vi "tStat2021_V3-19-04-2021.vi"() -> ()   [LabVIEW 2016]
doc: "This VI was designed to demonstrate typical usage of sub VIs containing the more common 335 functions. The VI Initializes the instrument, allows the user to determine if heater output control parameters and setpoint values are sent, takes a single sensor reading, and then closes the instrument."
uses:
  <instrlib>/Lake Shore 335/Public/Data/Sensor Data (Single Reading).vi
  <instrlib>/Lake Shore 335/Lake Shore 335.lvlib
panel:
  out "Ramping On":bool
  out "Ramping Active":bool
  out "Ramp Rate":dbl format="%.1f"
  out "Setpoint":dbl format="%.4f"
  in  "Ramp Rate (0.0)":dbl format="%.1f"
  in  "OK Button 2":bool
  in  "Mode 2":enum32{"Radio Selection 1", "Radio Selection 2"}(radio)
  in  "ШТОК 2":T1(radio)
  in  "Manual Output (0.00 %) 2":dbl format="%.2f"
  in  "Setpoint (0.0000) 2":dbl format="%.4f"
  out "x .and. y?":bool[](array[boolean])
  in  "Manual Output (0.00 %)":dbl format="%.2f"
  in  "Mode":enum32{"Radio Selection 1", "Radio Selection 2"}(radio)
  out "Температура в криоголовке":cluster{"Y":dbl[], "Y":dbl[]}[](graph)
  out "ТЕМПЕРАТУРА В КРИОГОЛОВКЕ":dbl format="%.4f"
  in  "Graph":bool
  out "Current":cluster{"Y":dbl[], "Y":dbl[]}[](graph)
  out "Temperature":cluster{"Y":dbl[], "Y":dbl[]}[](graph)
  in  "ШТОК":T1(radio)
  in  "Exit":bool
  out "Sensor Data":dbl format="%.4f"
  out "Heater power":dbl(graph)
  out "Temperature":dbl(graph)
  in  "Set":bool
  in  "Setpoint (0.0000)":dbl format="%.4f"
  # "Задать Ramping"
  # "Задавать при режиме Open Loop"
  # "Температуру на кpиоголовке"
  # "K/min"
  # "Температуру на кpиоголовке"
  # "(c) 2021 Vladimir Z Inc.  ALL RIGHTS RESERVED."
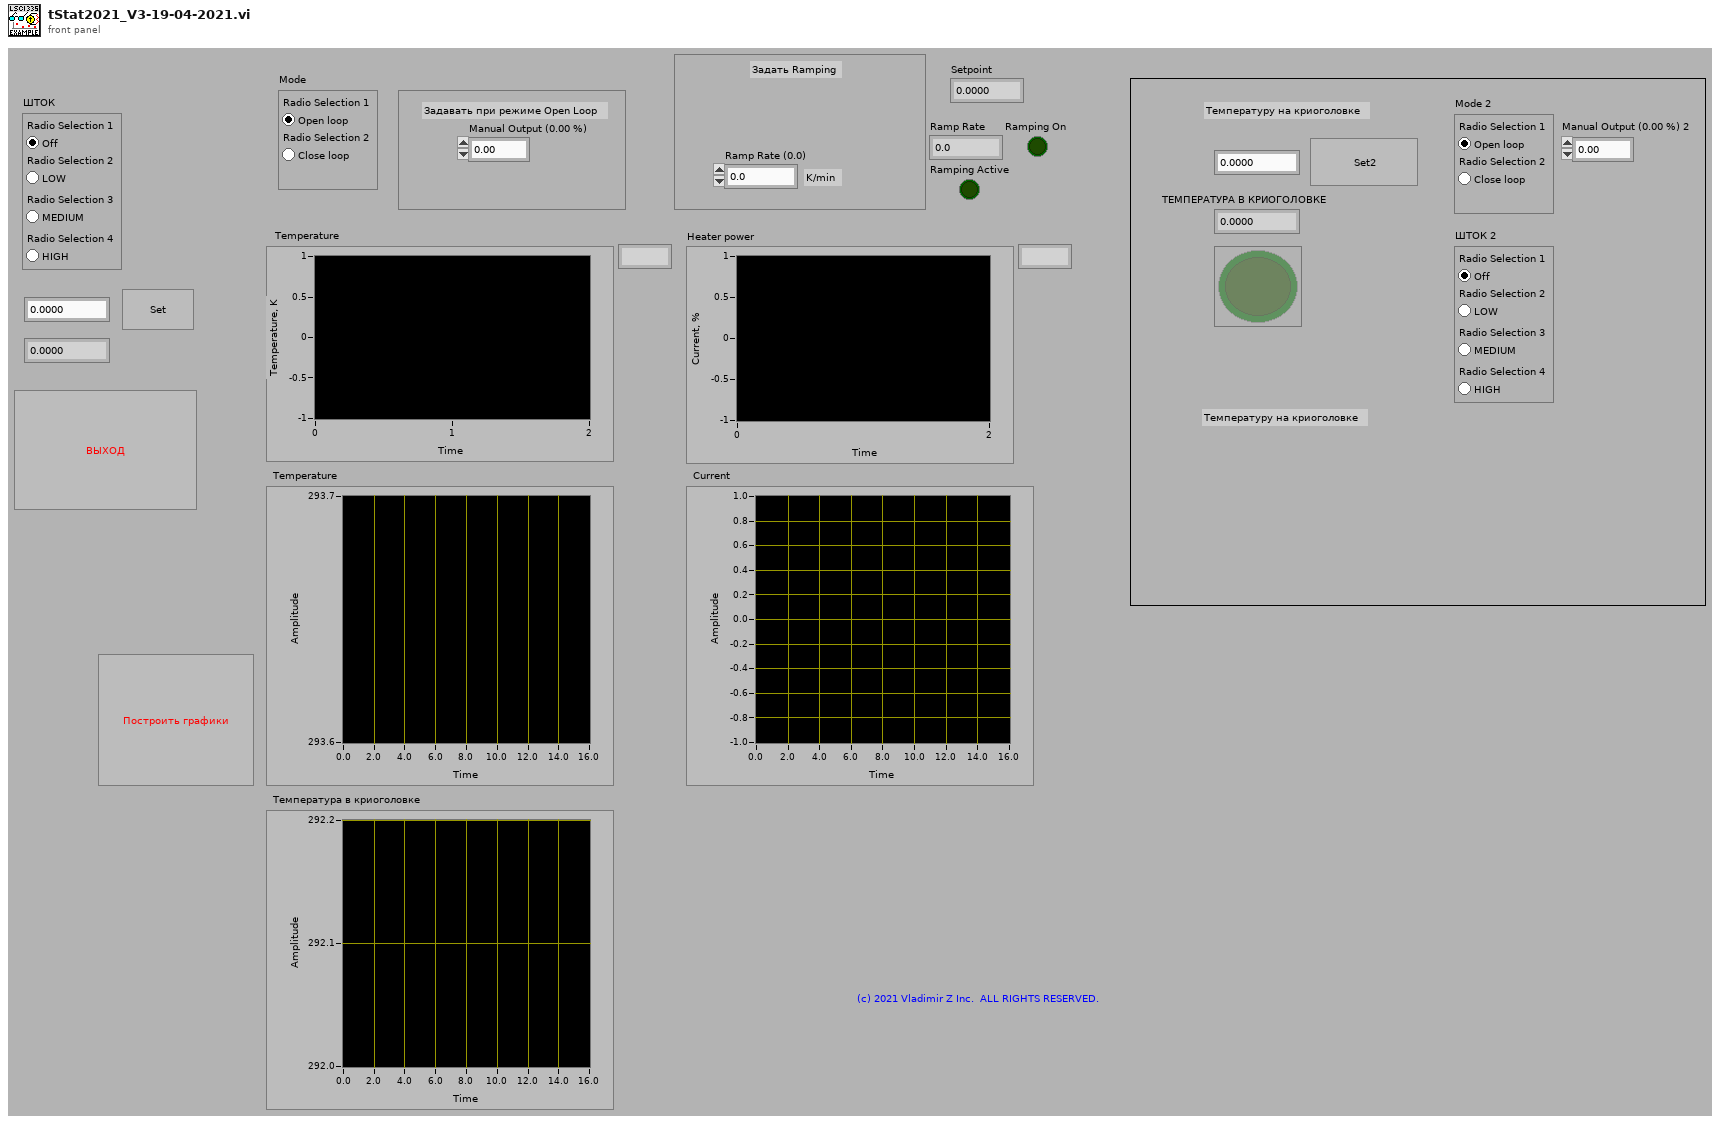
[diagram p1: front panel]
types:
  T1 = enum32{"Radio Selection 1", "Radio Selection 2", "Radio Selection 3", "Radio Selection 4"}
  T2 = cluster{"Baud Rate":u32, "Parity":u16, "Data Bits":u16, "Stop Bits":u16, "Flow Control":u16}
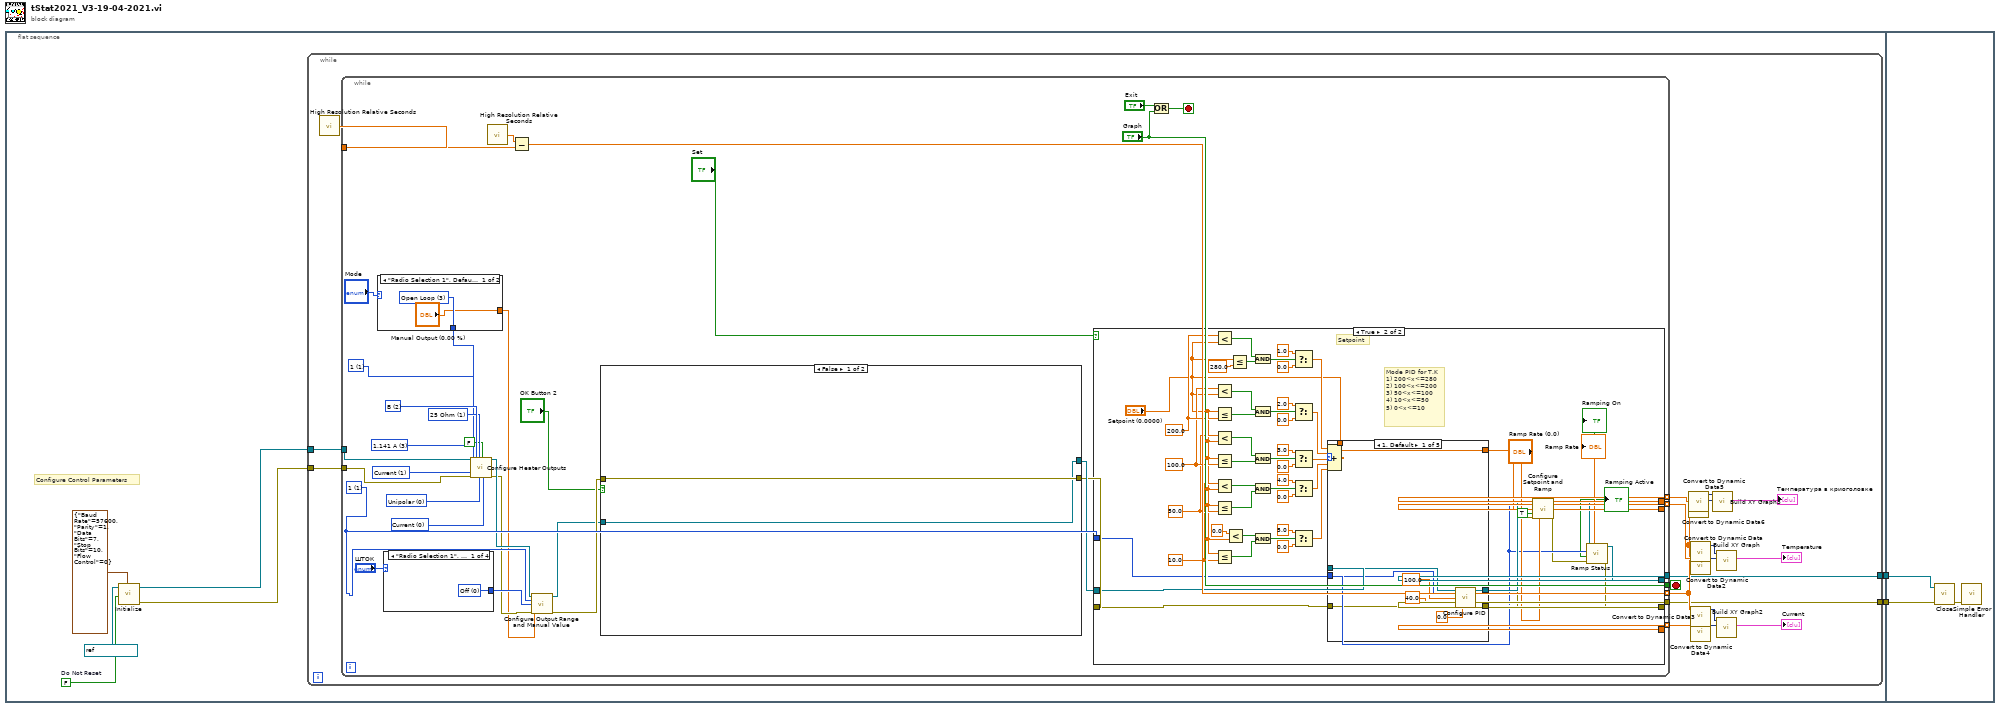
[diagram p0: block diagram]
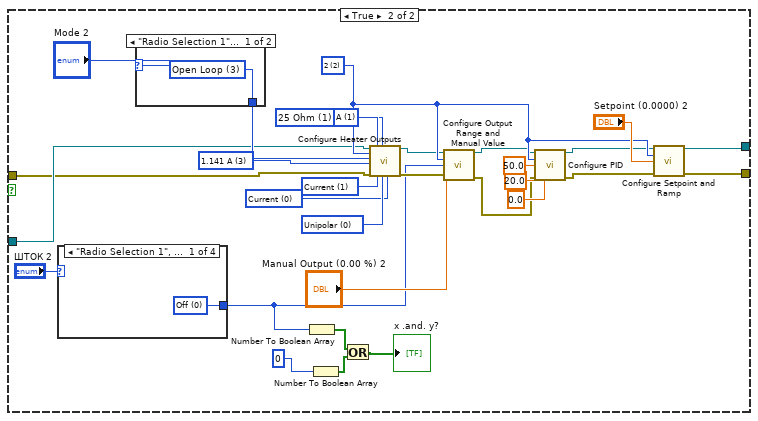
[diagram p2: hidden frame]
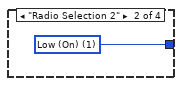
[diagram p3: hidden frame]
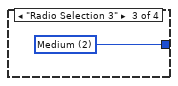
[diagram p4: hidden frame]
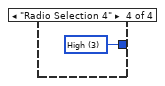
[diagram p5: hidden frame]
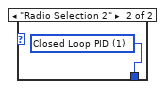
[diagram p6: hidden frame]
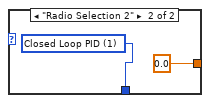
[diagram p7: hidden frame]
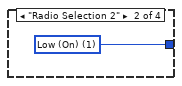
[diagram p8: hidden frame]
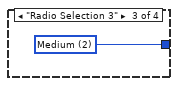
[diagram p9: hidden frame]
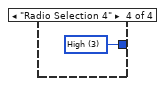
[diagram p10: hidden frame]
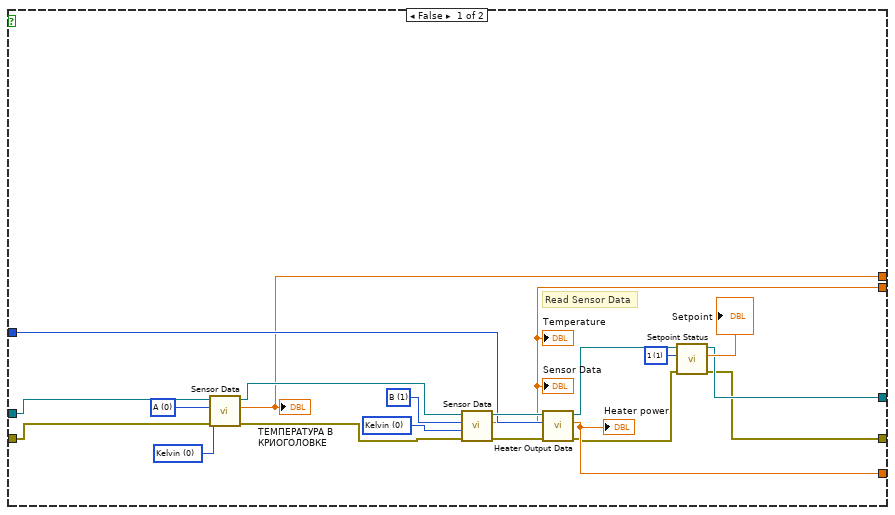
[diagram p11: hidden frame]
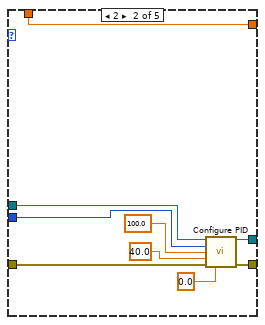
[diagram p12: hidden frame]
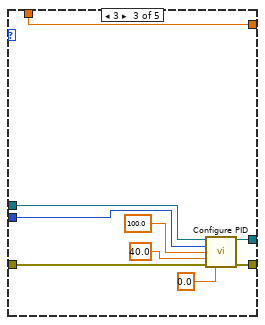
[diagram p13: hidden frame]
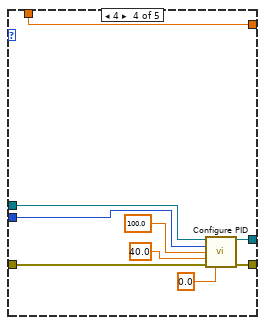
[diagram p14: hidden frame]
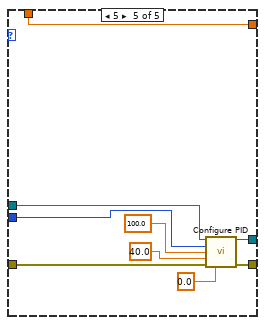
[diagram p15: hidden frame]
diagram:
  n1 = flat-sequence {
    tunnel: [w4] -> w2
    tunnel: [w3] -> w1
    tunnel: w2 -> [w229]
    tunnel: w1 -> [w228]
    frame #0 {
      w8 = FALSE  # Do Not Reset
      # "Configure Control Parameters"
      n2 = call <instrlib>:"Initialize.vi"("Serial Configuration"=T2 {"Baud Rate"=57600, "Parity"=1, "Data Bits"=7, "Stop Bits"=10, "Flow Control"=0}, "Reset (True)"=w8, "VISA resource name"=refnum<visa-resource-name> "Lakeshore") -> ("error out"=w5:errorcluster, "VISA resource name out"=w6:refnum<visa-resource-name>)  [unwired: 7 in]
      n3 = while {
        tunnel: w6 -> [w13]
        tunnel: w5 -> [w12]
        tunnel: [w11] -> w4
        tunnel: [w10] -> w3
        stop <- w20 stop-if-true
        n4 = call <vilib>:"High Resolution Relative Seconds.vi"() -> ("relative seconds"=w19:dbl)
        n5 = while {
          tunnel: [w62] -> w26 mode=indexing
          tunnel: [w61] -> w22 mode=indexing
          tunnel: w19 -> [w58]
          tunnel: [w57] -> w17 mode=indexing
          tunnel: ["Graph"] -> w20
          tunnel: [w53] -> w15 mode=indexing
          tunnel: w13 -> [w40]
          tunnel: w12 -> [w39]
          tunnel: [w38] -> w11
          tunnel: [w37] -> w10
          stop <- w55 stop-if-true
          w36 = u16 1 items=["1"=1, "2"=2] ("Heater Output (1:1)")
          w46 = u16 1 items=["25 Ohm"=1, "50 Ohm"=2] ("Heater Resistance (1:25 Ohm)")
          w47 = u16 2 items=["None", "A", "B"] ("Input (0:None)")
          w48 = u16 0 items=["Current", "Voltage"] ("Output Type (0:Current)")
          w49 = u16 0 items=["Unipolar", "Bipolar"] ("Polarity (0:Unipolar)")
          w50 = u16 1 items=["Current"=1, "Power"=2] ("Heater Out Display (1:Current)")
          w51 = u16 3 items=["User Specified", "0.707 A", "1.0 A", "1.141 A", "1.732 A"] ("Max Current (0:User Specified)")
          w52 = u16 1 items=["1"=1, "2"=2] ("Heater Output (1:1)")
          n6 = case shown="\"Radio Selection 1\", Default" "Mode" {
            tunnel: [w103 w105] -> w43
            tunnel: ["Manual Output (0.00 %)" 0.0 ("Manual Output (0.00 %)")] -> w29
            frame "Radio Selection 1", Default {
              w103 = u16 3 items=["Off", "Closed Loop PID", "Zone", "Open Loop", "Monitor Out", "Warmup Supply"] ("Mode (0:Off)")
            }
            frame "Radio Selection 2" {
              w105 = u16 1 items=["Off", "Closed Loop PID", "Zone", "Open Loop", "Monitor Out", "Warmup Supply"] ("Mode (0:Off)")
            }
          }
          n7 = case shown="\"Radio Selection 1\", Default" "ШТОК" {
            tunnel: [w106 w107 w108 w109] -> w60
            frame "Radio Selection 1", Default {
              w106 = u16 0 items=["Off", "Low (On)", "Medium", "High"] ("Range (0:Off)")
            }
            frame "Radio Selection 2" {
              w107 = u16 1 items=["Off", "Low (On)", "Medium", "High"] ("Range (0:Off)")
            }
            frame "Radio Selection 3" {
              w108 = u16 2 items=["Off", "Low (On)", "Medium", "High"] ("Range (0:Off)")
            }
            frame "Radio Selection 4" {
              w109 = u16 3 items=["Off", "Low (On)", "Medium", "High"] ("Range (0:Off)")
            }
          }
          n8 = call <instrlib>:"Configure Heater Outputs.vi"("VISA resource name"=w40, "Heater Output (1:1)"=w36, "Mode (0:Off)"=w43, "Max Current (0:User Specified)"=w51, "error in (no error)"=w39, "Input (0:None)"=w47, "Heater Out Display (1:Current)"=w50, "Heater Resistance (1:25 Ohm)"=w46, "Polarity (0:Unipolar)"=w49, "Power Up Enable (F: Off)"=FALSE, "Output Type (0:Current)"=w48) -> ("VISA resource name out"=w42:refnum<visa-resource-name>, "error out"=w41:errorcluster)  [unwired: 7 in]
          n9 = call <vilib>:"High Resolution Relative Seconds.vi"() -> ("relative seconds"=w59:dbl)
          n10 = Subtract(x=w59, y=w58) -> (x-y=w57:dbl)
          n11 = call <instrlib>:"Configure Output Range and Manual Value.vi"("VISA resource name"=w42, "Heater Output (1:1)"=w52, "Range (0:Off)"=w60, "Manual Output (0.00 %)"=w29, "error in (no error)"=w41) -> ("VISA resource name out"=w33:refnum<visa-resource-name>, "error out"=w34:errorcluster)  [unwired: 9 in]
          n12 = case shown="False" "OK Button 2" {
            tunnel: [w64 w74] -> w32
            tunnel: [w65 w73] -> w31
            tunnel: w33 -> [w64 w70]
            tunnel: w34 -> [w65 w69]
            frame False {
            }
            frame True {
              w88 = u16 1 items=["25 Ohm"=1, "50 Ohm"=2] ("Heater Resistance (1:25 Ohm)")
              w89 = u16 1 items=["None", "A", "B"] ("Input (0:None)")
              w90 = u16 0 items=["Current", "Voltage"] ("Output Type (0:Current)")
              w91 = u16 0 items=["Unipolar", "Bipolar"] ("Polarity (0:Unipolar)")
              w92 = u16 1 items=["Current"=1, "Power"=2] ("Heater Out Display (1:Current)")
              w93 = u16 3 items=["User Specified", "0.707 A", "1.0 A", "1.141 A", "1.732 A"] ("Max Current (0:User Specified)")
              w81 = u16 2 items=["1"=1, "2"=2] ("Heater Output (1:1)")
              n13 = case shown="\"Radio Selection 1\", Default" "ШТОК 2" {
                tunnel: [w96 w97 w98 w99] -> w72
                frame "Radio Selection 1", Default {
                  w96 = u16 0 items=["Off", "Low (On)", "Medium", "High"] ("Range (0:Off)")
                }
                frame "Radio Selection 2" {
                  w97 = u16 1 items=["Off", "Low (On)", "Medium", "High"] ("Range (0:Off)")
                }
                frame "Radio Selection 3" {
                  w98 = u16 2 items=["Off", "Low (On)", "Medium", "High"] ("Range (0:Off)")
                }
                frame "Radio Selection 4" {
                  w99 = u16 3 items=["Off", "Low (On)", "Medium", "High"] ("Range (0:Off)")
                }
              }
              n14 = case shown="\"Radio Selection 1\", Default" "Mode 2" {
                tunnel: [w100 w101] -> w94
                frame "Radio Selection 1", Default {
                  w100 = u16 3 items=["Off", "Closed Loop PID", "Zone", "Open Loop", "Monitor Out", "Warmup Supply"] ("Mode (0:Off)")
                }
                frame "Radio Selection 2" {
                  w101 = u16 1 items=["Off", "Closed Loop PID", "Zone", "Open Loop", "Monitor Out", "Warmup Supply"] ("Mode (0:Off)")
                }
              }
              n15 = Number To Boolean Array(number=w72) -> (Boolean array=w68:bool[])
              n16 = Number To Boolean Array(number=u16 0 ("y")) -> (Boolean array=w67:bool[])
              n17 = Or(x=w68, y=w67) -> (x .or. y?=→"x .and. y?":bool[])
              n18 = call <instrlib>:"Configure Heater Outputs.vi"("VISA resource name"=w70, "Heater Output (1:1)"=w81, "Mode (0:Off)"=w94, "Max Current (0:User Specified)"=w93, "error in (no error)"=w69, "Input (0:None)"=w89, "Heater Out Display (1:Current)"=w92, "Heater Resistance (1:25 Ohm)"=w88, "Polarity (0:Unipolar)"=w91, "Output Type (0:Current)"=w90) -> ("VISA resource name out"=w80:refnum<visa-resource-name>, "error out"=w79:errorcluster)  [unwired: 8 in]
              n19 = call <instrlib>:"Configure Output Range and Manual Value.vi"("VISA resource name"=w80, "Heater Output (1:1)"=w81, "Range (0:Off)"=w72, "Manual Output (0.00 %)"="Manual Output (0.00 %) 2", "error in (no error)"=w79) -> ("VISA resource name out"=w78:refnum<visa-resource-name>, "error out"=w77:errorcluster)  [unwired: 9 in]
              n20 = call <instrlib>:"Configure PID.vi"("VISA resource name"=w78, "Output's Control Loop (1:1)"=w81, "Gain (P) (50.0)"=50.0, "Reset (I) (20.0)"=20.0, "error in (no error)"=w77, "Rate (D) (0.0 %)"=0.0) -> ("VISA resource name out"=w76:refnum<visa-resource-name>, "error out"=w75:errorcluster)  [unwired: 8 in]
              n21 = call <instrlib>:"Configure Setpoint and Ramp.vi"("VISA resource name"=w76, "Output's Control Loop (1:1)"=w81, "Setpoint (0.0000)"="Setpoint (0.0000) 2", "error in (no error)"=w75) -> ("VISA resource name out"=w74:refnum<visa-resource-name>, "error out"=w73:errorcluster)  [unwired: 10 in]
            }
          }
          n22 = case shown="True" "Set" {
            tunnel: w32 -> [w122 w144]
            tunnel: w31 -> [w121 w145]
            tunnel: [w112 w132] -> w38
            tunnel: [w111 w131] -> w37
            tunnel: w52 -> [w126 w137]
            tunnel: [w124 _] -> w62
            tunnel: [w123 _] -> w61
            tunnel: [w116 _] -> w53
            frame False {
              w110 = u16 1 items=["1"=1, "2"=2] ("Output (1:1)")
              w117 = u16 0 items=["Kelvin", "Celsius", "Sensor Units"] ("Data Source (0:Kelvin)")
              w118 = u16 0 items=["A", "B"] ("Input (0:A)")
              w125 = u16 1 items=["A", "B"] ("Input (0:A)")
              w129 = u16 0 items=["Kelvin", "Celsius", "Sensor Units"] ("Data Source (0:Kelvin)")
              # "Read Sensor Data"
              n23 = call-poly <instrlib>:"Sensor Data.vi"("error in (no error)"=w121, "Data Source (0:Kelvin)"=w117, "Input (0:A)"=w118, "VISA resource name"=w122) -> ("error out"=w120:errorcluster, "Sensor Data"=w116:dbl, "VISA resource name out"=w119:refnum<visa-resource-name>)  [unwired: 5 in]
              "ТЕМПЕРАТУРА В КРИОГОЛОВКЕ" <- w116
              n24 = call-poly <instrlib>:"Sensor Data.vi"("error in (no error)"=w120, "Data Source (0:Kelvin)"=w129, "Input (0:A)"=w125, "VISA resource name"=w119) -> ("error out"=w127:errorcluster, "Sensor Data"=w124:dbl, "VISA resource name out"=w128:refnum<visa-resource-name>)  [unwired: 5 in]
              "Sensor Data" <- w124
              "Temperature" <- w124
              n25 = call <instrlib>:"Heater Output Data.vi"("error in (no error)"=w127, "Heater Output (1:1)"=w126, "VISA resource name"=w128) -> ("error out"=w115:errorcluster, "Output Value"=w123:dbl, "VISA resource name out"=w114:refnum<visa-resource-name>)  [unwired: 6 in]
              "Heater power" <- w123
              n26 = call <instrlib>:"Setpoint Status.vi"("error in (no error)"=w115, "Output (1:1)"=w110, "VISA resource name"=w114) -> ("error out"=w111:errorcluster, "Setpoint"=→"Setpoint":dbl, "VISA resource name out"=w112:refnum<visa-resource-name>)  [unwired: 6 in]
            }
            frame True {
              w147 = 10.0 ("x")
              w148 = 50.0 ("x")
              w149 = 100.0 ("x")
              w150 = 200.0 ("x")
              # "Mode PID for T,K\n1) 200<x<=280\n2) 100<x<=200\n3) 50<x<=100\n4) 10<x<=50\n5) 0<x<=10"
              # "Setpoint"
              n27 = Less?(x=w150, y="Setpoint (0.0000)") -> (x < y?=w153:bool)
              n28 = Less?(x=w149, y="Setpoint (0.0000)") -> (x < y?=w155:bool)
              n29 = Less Or Equal?(x="Setpoint (0.0000)", y=w150) -> (x <= y?=w154:bool)
              n30 = Less?(x=w148, y="Setpoint (0.0000)") -> (x < y?=w160:bool)
              n31 = Less Or Equal?(x="Setpoint (0.0000)", y=w149) -> (x <= y?=w161:bool)
              n32 = Less?(x=w147, y="Setpoint (0.0000)") -> (x < y?=w158:bool)
              n33 = Less Or Equal?(x="Setpoint (0.0000)", y=w148) -> (x <= y?=w159:bool)
              n34 = Less Or Equal?(x="Setpoint (0.0000)", y=w147) -> (x <= y?=w157:bool)
              n35 = Less?(x=0.0, y="Setpoint (0.0000)") -> (x < y?=w156:bool)
              n36 = Less Or Equal?(x="Setpoint (0.0000)", y=280.0 ("x")) -> (x <= y?=w152:bool)
              n37 = And(x=w153, y=w152) -> (x .and. y?=w169:bool)
              n38 = And(x=w155, y=w154) -> (x .and. y?=w163:bool)
              n39 = And(x=w160, y=w161) -> (x .and. y?=w164:bool)
              n40 = And(x=w158, y=w159) -> (x .and. y?=w166:bool)
              n41 = And(x=w156, y=w157) -> (x .and. y?=w165:bool)
              n42 = Select(t=1.0, s=w169, f=0.0) -> (s? t:f=w174:dbl)
              n43 = Select(t=2.0, s=w163, f=0.0) -> (s? t:f=w173:dbl)
              n44 = Select(t=3.0, s=w164, f=0.0) -> (s? t:f=w172:dbl)
              n45 = Select(t=4.0, s=w166, f=0.0) -> (s? t:f=w171:dbl)
              n46 = Select(t=5.0, s=w165, f=0.0) -> (s? t:f=w162:dbl)
              n47 = Compound Arithmetic op=ADD(w174, w173, w172, w171, w162) -> (w170:dbl)
              n48 = case shown="1, Default" w170 {
                tunnel: w137 -> [w191 w200 w209 w218 w227]
                tunnel: w144 -> [w187 w194 w205 w214 w220]
                tunnel: w145 -> [w186 w193 w204 w213 w223]
                tunnel: [w185 w196 w203 w212 w222] -> w143
                tunnel: [w184 w195 w202 w211 w221] -> w142
                tunnel: "Setpoint (0.0000)" -> [w183 w192 w201 w210 w219]
                tunnel: [w183 w192 w201 w210 w219] -> w140
                frame 1, Default {
                  n49 = call <instrlib>:"Configure PID.vi"("VISA resource name"=w187, "Output's Control Loop (1:1)"=w191, "Gain (P) (50.0)"=100.0, "Reset (I) (20.0)"=40.0, "error in (no error)"=w186, "Rate (D) (0.0 %)"=0.0) -> ("VISA resource name out"=w185:refnum<visa-resource-name>, "error out"=w184:errorcluster)  [unwired: 8 in]
                }
                frame 2 {
                  n50 = call <instrlib>:"Configure PID.vi"("VISA resource name"=w194, "Output's Control Loop (1:1)"=w200, "Gain (P) (50.0)"=100.0, "Reset (I) (20.0)"=40.0, "error in (no error)"=w193, "Rate (D) (0.0 %)"=0.0) -> ("VISA resource name out"=w196:refnum<visa-resource-name>, "error out"=w195:errorcluster)  [unwired: 8 in]
                }
                frame 3 {
                  n51 = call <instrlib>:"Configure PID.vi"("VISA resource name"=w205, "Output's Control Loop (1:1)"=w209, "Gain (P) (50.0)"=100.0, "Reset (I) (20.0)"=40.0, "error in (no error)"=w204, "Rate (D) (0.0 %)"=0.0) -> ("VISA resource name out"=w203:refnum<visa-resource-name>, "error out"=w202:errorcluster)  [unwired: 8 in]
                }
                frame 4 {
                  n52 = call <instrlib>:"Configure PID.vi"("VISA resource name"=w214, "Output's Control Loop (1:1)"=w218, "Gain (P) (50.0)"=100.0, "Reset (I) (20.0)"=40.0, "error in (no error)"=w213, "Rate (D) (0.0 %)"=0.0) -> ("VISA resource name out"=w212:refnum<visa-resource-name>, "error out"=w211:errorcluster)  [unwired: 8 in]
                }
                frame 5 {
                  n53 = call <instrlib>:"Configure PID.vi"("VISA resource name"=w220, "Output's Control Loop (1:1)"=w227, "Gain (P) (50.0)"=100.0, "Reset (I) (20.0)"=40.0, "error in (no error)"=w223, "Rate (D) (0.0 %)"=0.0) -> ("VISA resource name out"=w222:refnum<visa-resource-name>, "error out"=w221:errorcluster)  [unwired: 8 in]
                }
              }
              n54 = call <instrlib>:"Configure Setpoint and Ramp.vi"("VISA resource name"=w143, "Output's Control Loop (1:1)"=w137, "Setpoint (0.0000)"=w140, "Enable Setpoint Ramping (F: Off)"=TRUE, "error in (no error)"=w142, "Ramp Rate (0.0)"="Ramp Rate (0.0)") -> ("VISA resource name out"=w138:refnum<visa-resource-name>, "error out"=w133:errorcluster)  [unwired: 8 in]
              n55 = call <instrlib>:"Ramp Status.vi"("error in (no error)"=w133, "Output's Control Loop (1:1)"=w137, "VISA resource name"=w138) -> ("error out"=w131:errorcluster, "Ramping Active"=→"Ramping Active":bool, "Ramping On"=→"Ramping On":bool, "VISA resource name out"=w132:refnum<visa-resource-name>, "Ramp Rate"=→"Ramp Rate":dbl)  [unwired: 4 in]
            }
          }
          n56 = Or(x="Exit", y="Graph") -> (x .or. y?=w55:bool)
        }
        n57 = call "Convert to Dynamic Data5"("Array"=w17) -> ("Dynamic Data Type"=w16:dynamicdata)  [unwired: 3 in]
        n58 = call "Convert to Dynamic Data6"("Array"=w15) -> ("Dynamic Data Type"=w14:dynamicdata)  [unwired: 3 in]
        n59 = call "Convert to Dynamic Data"("Array"=w17) -> ("Dynamic Data Type"=w27:dynamicdata)  [unwired: 3 in]
        n60 = call "Convert to Dynamic Data2"("Array"=w26) -> ("Dynamic Data Type"=w25:dynamicdata)  [unwired: 3 in]
        n61 = call "Convert to Dynamic Data3"("Array"=w17) -> ("Dynamic Data Type"=w23:dynamicdata)  [unwired: 3 in]
        n62 = call "Convert to Dynamic Data4"("Array"=w22) -> ("Dynamic Data Type"=w21:dynamicdata)  [unwired: 3 in]
        n63 = call "Build XY Graph3"("Y Input"=w14, "X Input"=w16) -> ("XY Graph"=→"Температура в криоголовке":cluster{"X":dbl[], "Y":dbl[]}[])  [unwired: 8 in, 1 out]
        n64 = call "Build XY Graph"("Y Input"=w25, "X Input"=w27) -> ("XY Graph"=→"Temperature":cluster{"X":dbl[], "Y":dbl[]}[])  [unwired: 8 in, 1 out]
        n65 = call "Build XY Graph2"("Y Input"=w21, "X Input"=w23) -> ("XY Graph"=→"Current":cluster{"X":dbl[], "Y":dbl[]}[])  [unwired: 8 in, 1 out]
      }
    }
    frame #1 {
      n66 = call <instrlib>:"Close.vi"("error in (no error)"=w228, "VISA resource name"=w229) -> ("error out"=w230:errorcluster)  [unwired: 9 in]
      n67 = call <vilib>:"Simple Error Handler.vi"("error in (no error)"=w230) -> ()  [unwired: 4 in, 5 out]
    }
  }
